vi "Global 1.vi"() -> ()   [LabVIEW 2021]
panel:
  out "Array":bool[](array[boolean])
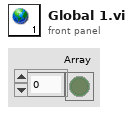
[diagram p1: front panel]
diagram:
